vi "CheckSync.vi"(9 "Current Time Stamp":timestamp, 10 "Remote Time Stamp":timestamp) -> (2 "Sync'd ?":bool)   [LabVIEW 2014]
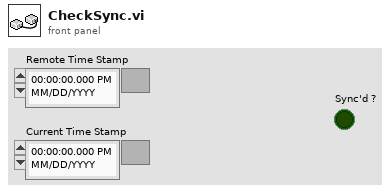
[diagram p1: front panel]
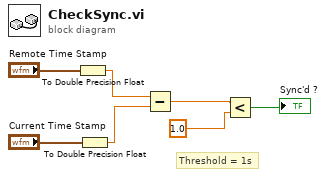
[diagram p0: block diagram]
diagram:
  # "Threshold = 1s"
  n1 = To Double Precision Float(number="Remote Time Stamp") -> (double precision float=w5:dbl)
  n2 = To Double Precision Float(number="Current Time Stamp") -> (double precision float=w4:dbl)
  n3 = Subtract(x=w5, y=w4) -> (x-y=w3:dbl)
  n4 = Less?(x=w3, y=1.0) -> (x < y?=→"Sync'd ?":bool)
